vi "Regenerate gRPC code.vi"(8 "error in (no error)":errorcluster, 11 "proto File Path":path) -> (0 "error out":errorcluster)   [LabVIEW 2021, in "TemplateCoreUtilities.lvlib"]
uses:
  TemplateCoreUtilities.lvlib
panel:
  # "Instructions:\nIf run from the default location the proto file path can be left empty and it will auto-detect the path.  \nRun the VI.  It will attempt to generate and replace the existing gRPC server and client code."
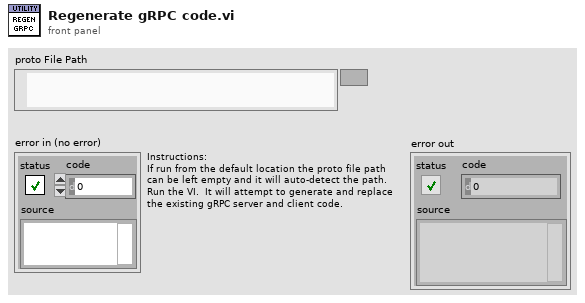
[diagram p1: front panel]
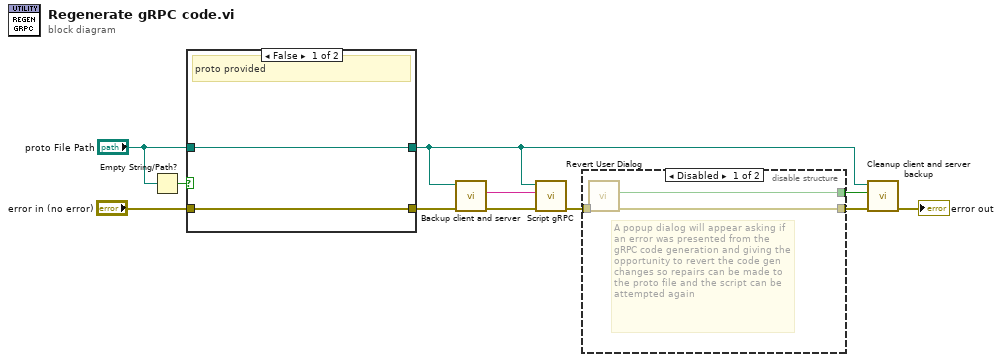
[diagram p0: block diagram]
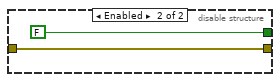
[diagram p2: hidden frame]
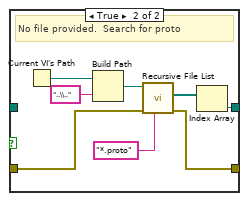
[diagram p3: hidden frame]
diagram:
  n1 = Empty String/Path?(string/path="proto File Path") -> (empty?=w6:bool)
  n2 = case shown="False" w6 {
    tunnel: [w12 w17] -> w8
    tunnel: [w13 w15] -> w5
    tunnel: "proto File Path" -> [w13 _]
    tunnel: "error in (no error)" -> [w12 w14]
    frame False {
      # "proto provided"
    }
    frame True {
      # "No file provided.  Search for proto"
      n3 = Current VI's Path() -> (path=w20:path)
      n4 = Build Path(base path=w20, name or relative path="..\\.." ("String")) -> (appended path=w19:path)
      n5 = call <vilib>:"Recursive File List.vi"("pattern"="*.proto", "error in (no error)"=w14, "Folder Path"=w19) -> ("error out"=w17:errorcluster, "All Files in Dir"=w16:path[])  [unwired: 4 in, 3 out]
      n6 = Index Array(array=w16) -> (element=w15:path)  [unwired: 1 in]
    }
  }
  n7 = call "Backup client and server.vi"("error in"=w8, "proto File Path"=w5) -> ("error out"=w11:errorcluster, "Generated Library Name"=w10:string)  [unwired: 8 in]
  n8 = call "Script gRPC.vi"("error in"=w11, "Generated Library Name"=w10, "proto File Path"=w5) -> ("error out"=w4:errorcluster)  [unwired: 8 in]
  n9 = disable-structure shown="Disabled" {
    disable-tunnel: w4 -> [w24 w26]
    disable-tunnel: [w23 w26] -> w3
    disable-tunnel: [w22 FALSE ("Revert")] -> w2
    frame Disabled {
      # "A popup dialog will appear asking if an error was presented from the gRPC code generation and giving the opportunity to revert the code gen changes so repairs can be made to the proto file and the script can be attempted again"
      n10 = call "Revert User Dialog.vi"("error in (no error)"=w24) -> ("error out"=w23:errorcluster, "Revert"=w22:bool)  [unwired: 9 in]
    }
    frame Enabled {
    }
  }
  n11 = call "Cleanup client and server backup.vi"("error in"=w3, "Revert"=w2, "proto File Path"=w5) -> ("error out"=→"error out":errorcluster)  [unwired: 8 in]
